vi "Close_VIs.vi"(8 "error in":errorcluster) -> (0 "error out":errorcluster, 3 "State Out":T1)   [LabVIEW 2019]
uses:
  #typedef_Controller_Action_enum.ctl
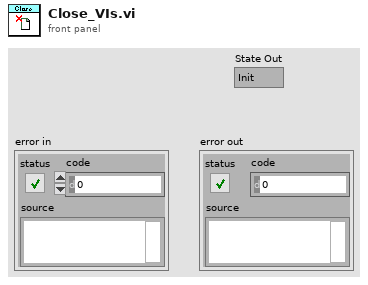
[diagram p1: front panel]
types:
  T1 = typedef "#typedef_Controller_Action_enum.ctl" = enum16{"Init", "ERROR_DEFAULT", "Idle", "Read database", "Close", "Error_Handler", "Exit"}
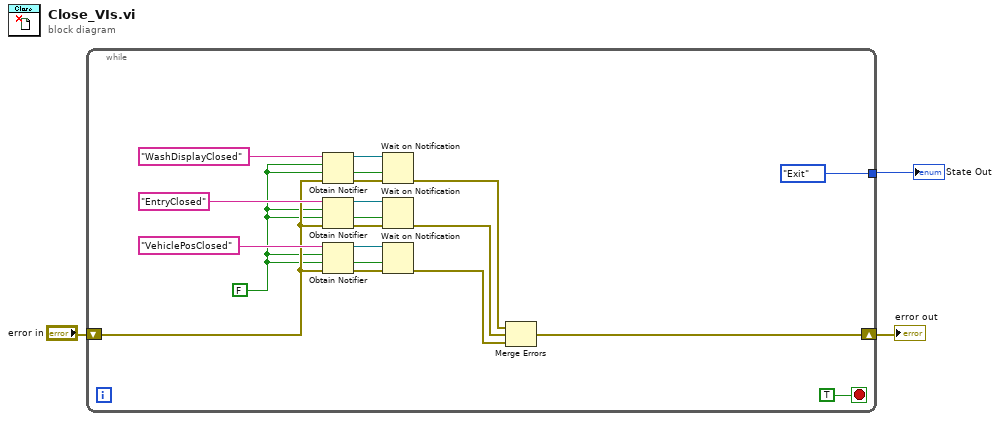
[diagram p0: block diagram]
diagram:
  n1 = while {
    tunnel: [#typedef_Controller_Action_enum."Exit" ("Enum")] -> w1
    shift-right: [w6] -> w3
    shift-left: "error in" -> [w5]
    stop <- TRUE stop-if-true
    w4 = FALSE ("create if not found? (T)")
    n2 = Obtain Notifier(name (unnamed)="WashDisplayClosed", notification data type=w4, create if not found? (T)=w4, error in (no error)=w5) -> (notifier out=w22:refnum<notifier>, created new?=w21:bool, error out=w20:errorcluster)
    n3 = Obtain Notifier(name (unnamed)="EntryClosed", notification data type=w4, create if not found? (T)=w4, error in (no error)=w5) -> (notifier out=w16:refnum<notifier>, created new?=w17:bool, error out=w18:errorcluster)
    n4 = Obtain Notifier(name (unnamed)="VehiclePosClosed", notification data type=w4, create if not found? (T)=w4, error in (no error)=w5) -> (notifier out=w15:refnum<notifier>, created new?=w14:bool, error out=w13:errorcluster)
    n5 = Wait on Notification(notifier=w22, ignore previous (F)=w21, error in (no error)=w20) -> (error out=w9:errorcluster)  [unwired: 1 in, 3 out]
    n6 = Wait on Notification(notifier=w16, ignore previous (F)=w17, error in (no error)=w18) -> (error out=w8:errorcluster)  [unwired: 1 in, 3 out]
    n7 = Wait on Notification(notifier=w15, ignore previous (F)=w14, error in (no error)=w13) -> (error out=w7:errorcluster)  [unwired: 1 in, 3 out]
    n8 = Merge Errors(w9, w8, w7) -> (w6:errorcluster)
  }
  "error out" <- w3
  "State Out" <- w1
